vi "PiLoN_data_processor.vi"(8 "PumpOffBkgd":dbl[](array[numeric]), 9 "PumpOnBkgd":dbl[](array[numeric]), 10 "Data":dbl[][](array[numeric]), 11 "# of Images":u16) -> (0 "Pump_Off":dbl[](array[numeric]), 1 "Pump_On":dbl[](array[numeric]), 2 "Raman_Gain":dbl[](array[numeric]))   [LabVIEW 2015]
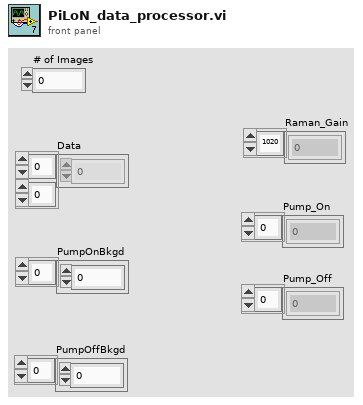
[diagram p1: front panel]
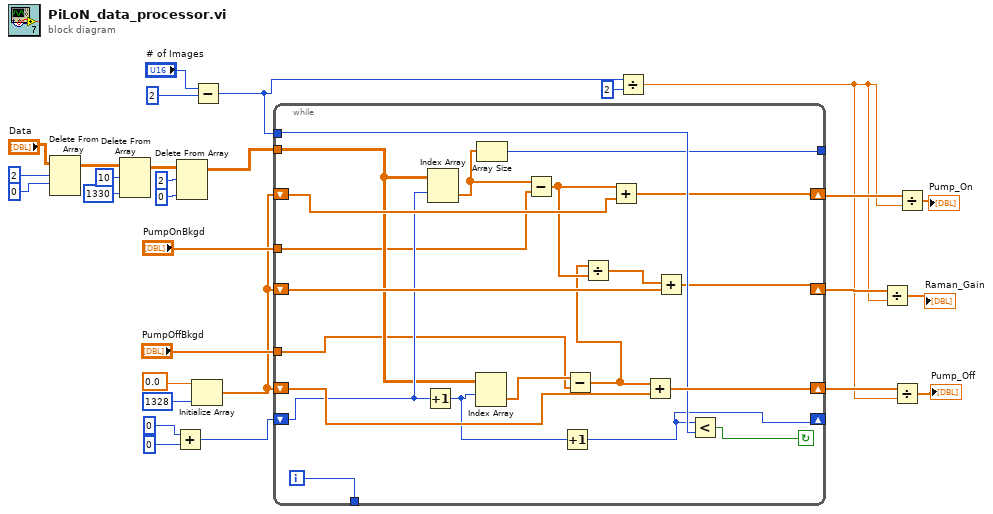
[diagram p0: block diagram]
diagram:
  n1 = Delete From Array(array="Data", length=2, index (row)=0 ("disabled index (col)")) -> (array with subset deleted=w9:dbl[][])  [unwired: 1 in, 1 out]
  n2 = Delete From Array(array=w9, length=10, index (col)=1330 ("disabled index (col)")) -> (array with subset deleted=w6:dbl[][])  [unwired: 1 in, 1 out]
  n3 = Add(x=0, y=0) -> (x+y=w18:i32)
  n4 = Delete From Array(array=w6, length=2, index (col)=0 ("disabled index (col)")) -> (array with subset deleted=w3:dbl[][])  [unwired: 1 in, 1 out]
  n5 = Initialize Array(0.0, u32 1328) -> (w2:dbl[])
  n6 = Subtract(x="# of Images", y=2) -> (x-y=w15:i32)
  n7 = while {
    tunnel: w3 -> [w35]
    shift-right: [w41] -> w14
    shift-left: w2 -> [w48]
    shift-right: [w49] -> w28
    shift-left: w2 -> [w50]
    tunnel: w15 -> [w47]
    shift-right: [w40] -> w24
    shift-left: w2 -> [w46]
    shift-right: [w30] -> _
    shift-left: w18 -> [w42]
    tunnel: "PumpOnBkgd" -> [w34]
    tunnel: "PumpOffBkgd" -> [w33]
    tunnel: [w39] -> _
    tunnel: [w36] -> _
    i -> [w36]
    stop <- w45 continue-if-true
    n8 = Increment(x=w42) -> (x+1=w31:i32)
    n9 = Index Array(array=w35, index (row)=w42) -> (element=w38:dbl[])  [unwired: 1 in]
    n10 = Index Array(array=w35, index (row)=w31) -> (element=w37:dbl[])  [unwired: 1 in]
    n11 = Array Size(array=w38) -> (size(s)=w39:i32)
    n12 = Subtract(x=w38, y=w34) -> (x-y=w44:dbl[])
    n13 = Increment(x=w31) -> (x+1=w30:i32)
    n14 = Subtract(x=w37, y=w33) -> (x-y=w43:dbl[])
    n15 = Divide(x=w43, y=w44) -> (x/y=w32:dbl[])
    n16 = Add(x=w44, y=w48) -> (x+y=w41:dbl[])
    n17 = Add(x=w43, y=w50) -> (x+y=w49:dbl[])
    n18 = Add(x=w32, y=w46) -> (x+y=w40:dbl[])
    n19 = Less?(x=w30, y=w47) -> (x < y?=w45:bool)
  }
  n20 = Divide(x=w15, y=2) -> (x/y=w1:dbl)
  n21 = Divide(x=w24, y=w1) -> (x/y=→"Raman_Gain":dbl[])
  n22 = Divide(x=w28, y=w1) -> (x/y=→"Pump_Off":dbl[])
  n23 = Divide(x=w14, y=w1) -> (x/y=→"Pump_On":dbl[])
